vi "Current to Field Converter.vi"(1 "Field constant [T/A]":dbl, 2 "Current in [A]":dbl) -> (0 "Field out [T]":dbl)   [LabVIEW 2022 SP3, in "Magnet module.lvlib"]
doc: "Params: \nCurrent in - current thought coil\nField constant - conversion constant (tesla per amper)\nReturn:\nField out - Magnetic field inside a coil"
uses:
  Magnet module.lvlib
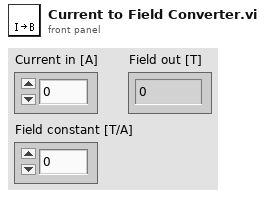
[diagram p1: front panel]
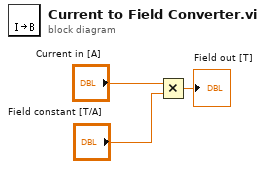
[diagram p0: block diagram]
diagram:
  n1 = Multiply(x="Current in [A]", y="Field constant [T/A]") -> (x*y=→"Field out [T]":dbl)
